vi "FlagInstance-CSMKVMap.vi"(10 "Error in":errorcluster caption="Error in (no error)") -> (2 "Error out":errorcluster, 3 "Changed":bool)   [LabVIEW 2017, in "Communicable State Machine.lvlib"]
uses:
  Communicable State Machine.lvlib
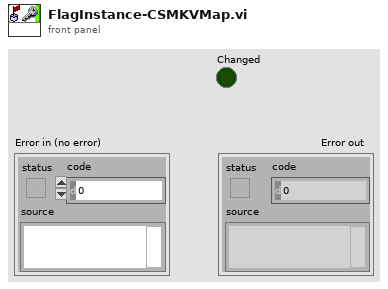
[diagram p1: front panel]
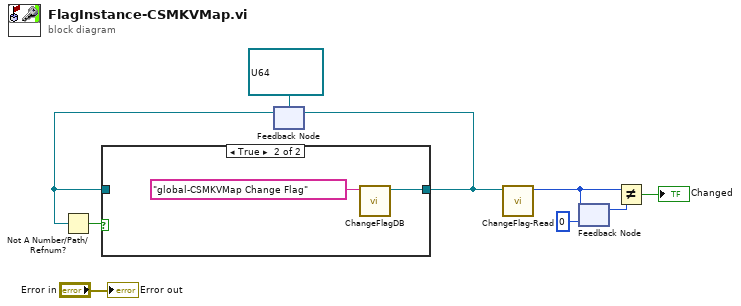
[diagram p0: block diagram]
diagram:
  n1 = feedback #1(refnum<queue> refnum ("ChangeFlagQ")) -> (w7:refnum<queue>)
  n2 = Not A Number/Path/Refnum?(number/path/refnum=w7) -> (NaN/Path/Refnum?=w8:bool)
  n3 = case shown="True" w8 {
    tunnel: [w10 w11] -> w6
    tunnel: w7 -> [w10 _]
    frame False {
    }
    frame True {
      n4 = call "ChangeFlagDB.vi"("ChangeFlagName"="global-CSMKVMap Change Flag" ("global-CSMQ FGV Change Flag")) -> ("ChangeFlagQ"=w11:refnum<queue>)  [unwired: 10 in]
    }
  }
  n5 = feedback-in #1(w6) -> ()
  n6 = call "ChangeFlag-Read.vi"("ChangeFlagQ"=w6) -> ("ChangeFlag"=w4:u64)  [unwired: 9 in, 1 out]
  n7 = feedback #2(u64 0 ("ChangeFlag")) -> (w5:u64)
  n8 = feedback-in #2(w4) -> ()
  n9 = Not Equal?(x=w4, y=w5) -> (x != y?=→"Changed":bool)
  "Error out" <- "Error in"
